vi "Animation 2D.vi"(0 "m2":dbl(knob)=6.0 scale=90.0..-90.0, 1 "m3":dbl(knob)=6.0 scale=90.0..-90.0, 2 "m5":dbl(knob)=6.0 scale=90.0..-90.0, 3 "m6":dbl(knob)=6.0 scale=90.0..-23.0, 4 "error in (no error)":errorcluster) -> (7 "Picture":picture, 10 "error out":errorcluster)   [LabVIEW 2017]
doc: "This VI animates a robotic arm using a 2D Picture. By changing the knobs and sliders, you can change the lengths and angles of the various components of the arm."
panel:
  in  "Scale Factor":dbl(slide)=0.7 scale=0.5..1.0
  in  "Light Direction":dbl(knob)=5.611498737356196 scale format="%#.1f"
  in  "Add details":bool=TRUE
  in  "Colors":T1={"m2"=16750848, "Arm A"=16764006, "m3"=26316, "Arm B"=6723993, "Joint C"=16724787, "m6"=16776960, "Joint D"=26316, "Arm Y"=6723993, "m5"=26316, "Arm J"=6723993}
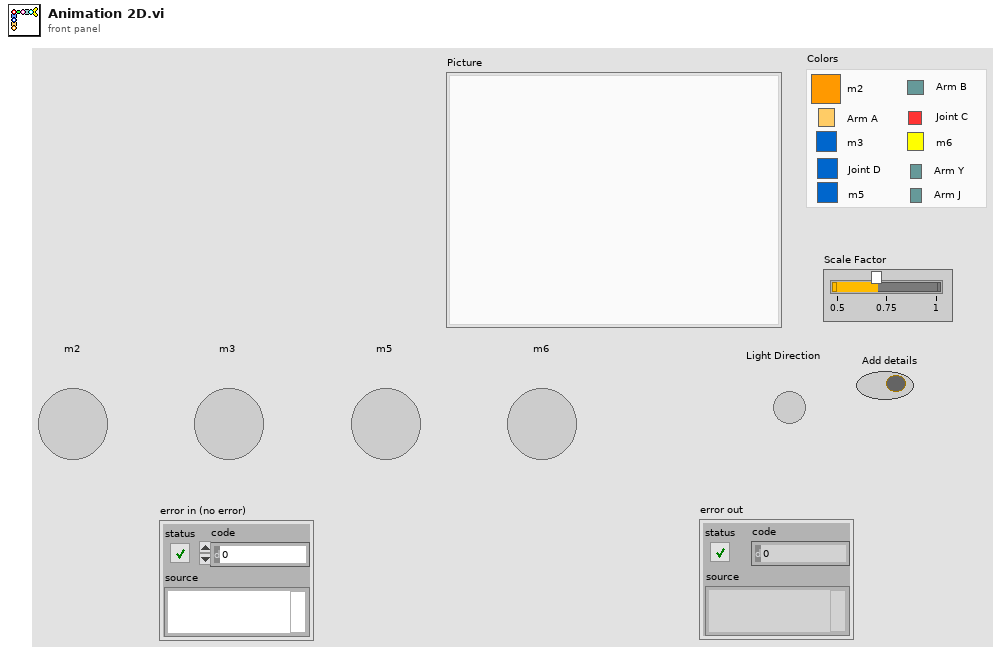
[diagram p1: front panel]
types:
  T1 = cluster{"m2":u32, "Arm A":u32, "m3":u32, "Arm B":u32, "Joint C":u32, "m6":u32, "Joint D":u32, "Arm Y":u32, "m5":u32, "Arm J":u32}
  T2 = cluster{"top":dbl, "left":dbl, "height":dbl, "width":dbl}
  T3 = cluster{"left":dbl, "top":dbl, "right":dbl, "bottom":dbl}
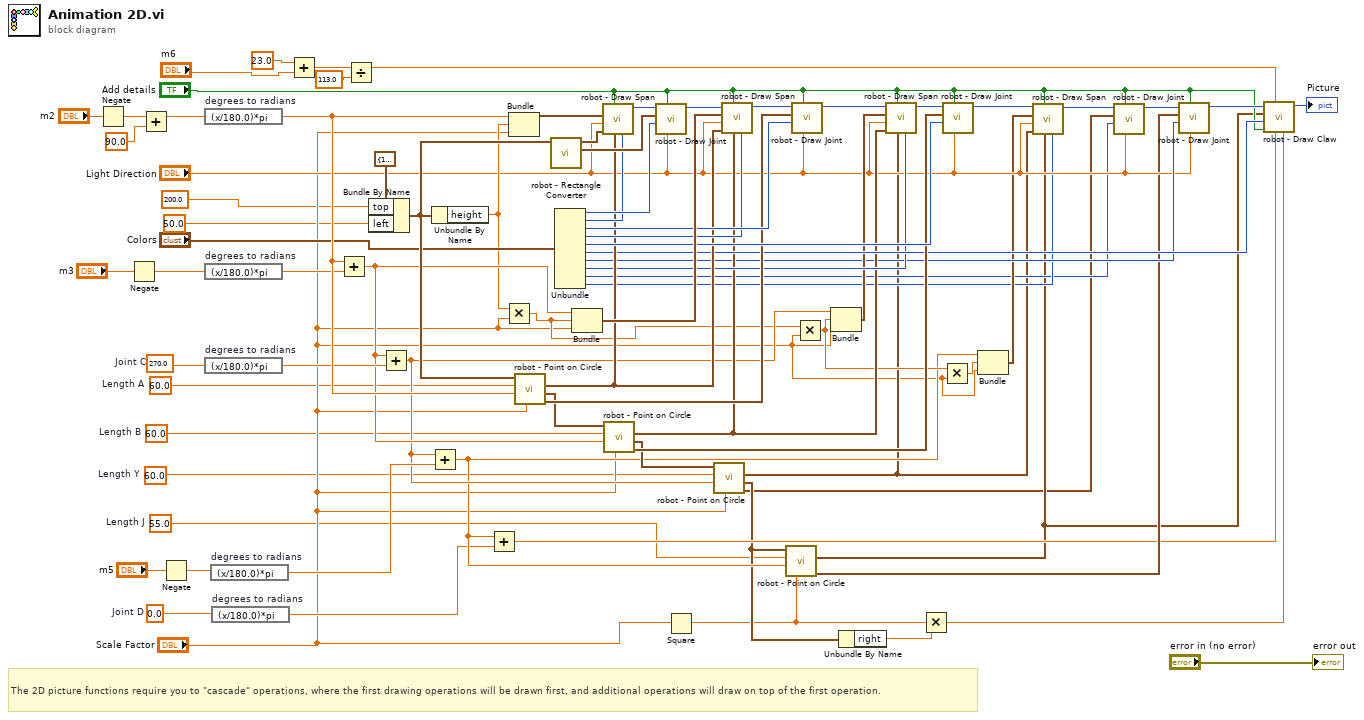
[diagram p0: block diagram]
diagram:
  w14 = 0.0  # Joint D
  w15 = 55.0  # Length J
  w16 = 60.0  # Length Y
  w17 = 60.0  # Length B
  w18 = 60.0  # Length A
  w19 = 270.0  # Joint C
  # "The 2D picture functions require you to \"cascade\" operations, where the first drawing operations will be drawn first, and additional operations will draw on top of the first operation."
  n1 = Negate(x="m2") -> (-x=w7:dbl)
  n2 = Negate(x="m3") -> (-x=w6:dbl)
  n3 = Add(x=w7, y=90.0) -> (x+y=w13:dbl)
  n4 = Negate(x="m5") -> (-x=w5:dbl)
  n5 = expression code="(x/180.0)*pi" "degrees to radians"(w13) -> (w67:dbl)
  n6 = expression code="(x/180.0)*pi" "degrees to radians"(w6) -> (w64:dbl)
  n7 = expression code="(x/180.0)*pi" "degrees to radians"(w19) -> (w66:dbl)
  n8 = expression code="(x/180.0)*pi" "degrees to radians"(w5) -> (w48:dbl)
  n9 = expression code="(x/180.0)*pi" "degrees to radians"(w14) -> (w22:dbl)
  n10 = Add(x=23.0, y="m6") -> (x+y=w11:dbl)
  n11 = Add(x=w67, y=w64) -> (x+y=w53:dbl)
  n12 = Divide(x=w11, y=113.0) -> (x/y=w9:dbl)
  n13 = Bundle By Name(cluster=T2 {"top"=120.0, "left"=70.0, "height"=32.0, "width"=32.0} ("Circle"), "top"=200.0 ("Base position Y"), "left"=50.0) -> (w63:T2)
  n14 = Add(x=w53, y=w66) -> (x+y=w44:dbl)
  n15 = Add(x=w44, y=w48) -> (x+y=w27:dbl)
  n16 = Unbundle By Name(w63) -> ("height"=w47:dbl)
  n17 = Add(x=w27, y=w22) -> (x+y=w31:dbl)
  n18 = Multiply(x=w47, y="Scale Factor") -> (x*y=w40:dbl)
  n19 = Bundle(w67, "height"=w47, "Scale Factor"="Scale Factor") -> (w79:cluster{dbl, "height":dbl, "Scale Factor":dbl})  [unwired: 1 in]
  n20 = call "robot - Point on Circle.vi"("Scale Factor"="Scale Factor", "Angle"=w67, "Radius"=w18, "Rect In"=w63) -> ("Scaled Rect Out"=w59:T3, "Rect Out"=w58:T3, "scaled point"=w60:cluster{"x":dbl, "y":dbl})  [unwired: 4 in, 1 out]
  n21 = call "robot - Rectangle Converter.vi"("Rect"=w63) -> ("Rect Out"=w73:T3, "Center"=w62:cluster{"x":dbl, "y":dbl})  [unwired: 9 in]
  n22 = Unbundle("Colors") -> ("m2"=w74:u32, "Arm A"=w71:u32, "m3"=w75:u32, "Arm B"=w70:u32, "Joint C"=w76:u32, "m6"=w55:u32, "Joint D"=w42:u32, "Arm Y"=w52:u32, "m5"=w28:u32, "Arm J"=w29:u32)
  n23 = Bundle(w53, w40, "Scale Factor"="Scale Factor") -> (w80:cluster{dbl, dbl, "Scale Factor":dbl})  [unwired: 1 in]
  n24 = call "robot - Draw Span.vi"("Color"=w71, "Center 2"=w60, "Enhance Style"="Add details", "Center 1"=w62, "Light Direction"="Light Direction", "Circle Spec"=w79) -> ("Picture Out"=w77:picture)  [unwired: 5 in]
  n25 = call "robot - Point on Circle.vi"("Scale Factor"="Scale Factor", "Angle"=w53, "Radius"=w17, "Rect In"=w58) -> ("Scaled Rect Out"=w61:T3, "Rect Out"=w41:T3, "scaled point"=w46:cluster{"x":dbl, "y":dbl})  [unwired: 4 in, 1 out]
  n26 = call "robot - Draw Joint.vi"("Light Direction"="Light Direction", "Enhance Style"="Add details", "Color"=w74, "Rectangle"=w73, "Picture In"=w77) -> ("Picture Out"=w57:picture)  [unwired: 6 in]
  n27 = Square(x="Scale Factor") -> (x^2=w20:dbl)
  n28 = call "robot - Point on Circle.vi"("Scale Factor"="Scale Factor", "Angle"=w44, "Radius"=w16, "Rect In"=w41) -> ("Scaled Rect Out"=w24:T3, "Rect Out"=w26:T3, "scaled point"=w23:cluster{"x":dbl, "y":dbl})  [unwired: 4 in, 1 out]
  n29 = call "robot - Draw Span.vi"("Color"=w70, "Center 2"=w46, "Enhance Style"="Add details", "Center 1"=w60, "Light Direction"="Light Direction", "Circle Spec"=w80, "Picture In"=w57) -> ("Picture Out"=w78:picture)  [unwired: 4 in]
  n30 = call "robot - Point on Circle.vi"("Scale Factor"=w20, "Angle"=w27, "Radius"=w15, "Rect In"=w26) -> ("Scaled Rect Out"=w32:T3, "scaled point"=w25:cluster{"x":dbl, "y":dbl})  [unwired: 4 in, 2 out]
  n31 = call "robot - Draw Joint.vi"("Light Direction"="Light Direction", "Enhance Style"="Add details", "Color"=w75, "Rectangle"=w59, "Picture In"=w78) -> ("Picture Out"=w51:picture)  [unwired: 6 in]
  n32 = Multiply(x=w40, y="Scale Factor") -> (x*y=w30:dbl)
  n33 = Bundle(w44, w30, "Scale Factor"="Scale Factor") -> (w50:cluster{dbl, dbl, "Scale Factor":dbl})  [unwired: 1 in]
  n34 = Unbundle By Name(w26) -> ("right"=w72:dbl)
  n35 = call "robot - Draw Span.vi"("Color"=w52, "Center 2"=w23, "Enhance Style"="Add details", "Center 1"=w46, "Light Direction"="Light Direction", "Circle Spec"=w50, "Picture In"=w51) -> ("Picture Out"=w45:picture)  [unwired: 4 in]
  n36 = Multiply(x=w20, y=w72) -> (x*y=w56:dbl)
  n37 = Multiply(x=w30, y="Scale Factor") -> (x*y=w38:dbl)
  n38 = call "robot - Draw Joint.vi"("Light Direction"="Light Direction", "Enhance Style"="Add details", "Color"=w76, "Rectangle"=w61, "Picture In"=w45) -> ("Picture Out"=w37:picture)  [unwired: 6 in]
  n39 = Bundle(w27, w38, "Scale Factor"="Scale Factor") -> (w33:cluster{dbl, dbl, "Scale Factor":dbl})  [unwired: 1 in]
  n40 = call "robot - Draw Span.vi"("Color"=w29, "Center 2"=w25, "Enhance Style"="Add details", "Center 1"=w23, "Light Direction"="Light Direction", "Circle Spec"=w33, "Picture In"=w37) -> ("Picture Out"=w39:picture)  [unwired: 4 in]
  n41 = call "robot - Draw Joint.vi"("Light Direction"="Light Direction", "Enhance Style"="Add details", "Color"=w28, "Rectangle"=w24, "Picture In"=w39) -> ("Picture Out"=w36:picture)  [unwired: 6 in]
  n42 = call "robot - Draw Joint.vi"("Light Direction"="Light Direction", "Enhance Style"="Add details", "Color"=w42, "Rectangle"=w32, "Picture In"=w36) -> ("Picture Out"=w43:picture)  [unwired: 6 in]
  n43 = call "robot - Draw Claw.vi"("Diameter"=w56, "Claw Angle"=w31, "Claw Value"=w9, "Enhance Style"="Add details", "Claw Color"=w55, "Position"=w25, "Picture In"=w43) -> ("Picture Out"=→"Picture":picture)  [unwired: 4 in]
  "error out" <- "error in (no error)"
